vi "Read I16 analogue Data.vi"(6 "Block Header":string, 7 "Channel info":T1[](array[typedef]), 8 "Time Trace In":T2[](array[typedef]), 9 "Anaologue Index":i32[](array[numeric]), 10 "pos offset (bytes:0)":i32, 11 "refnum":refnum<file>) -> (0 "Time Trace out":T2[](array[typedef]), 1 "EOF?":bool, 2 "mark after read (bytes)":i32)   [LabVIEW 2017]
uses:
  Controls/Time_Trace_Cluster.ctl
  Controls/Read I16 data cluster.ctl
  Globals/Meas_global.vi
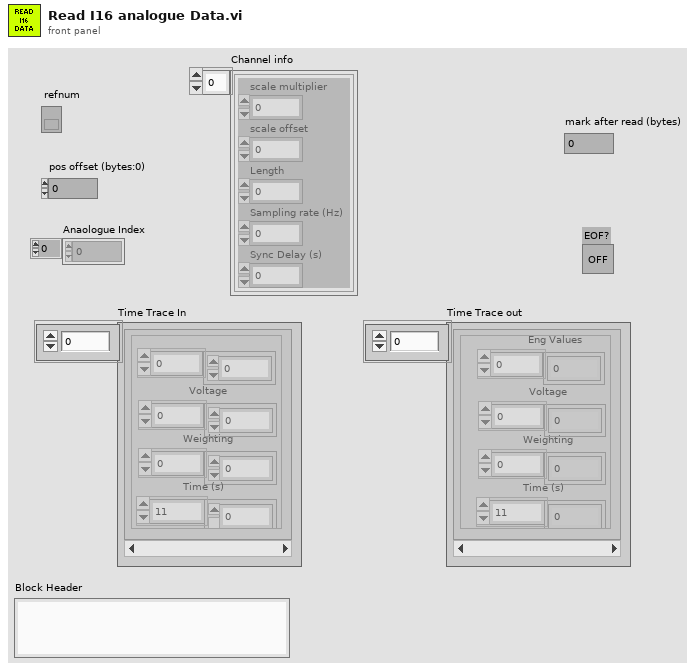
[diagram p1: front panel]
types:
  T1 = typedef "Read I16 data cluster.ctl" = cluster{"scale multiplier":dbl, "scale offset":dbl, "Length":i32, "Sampling rate (Hz)":dbl, "Sync Delay (s)":dbl}
  T2 = typedef "Time_Trace_Cluster.ctl" = cluster{"Weighting":dbl[], "Time (s)":dbl[], "Voltage":dbl[], "Eng Values":dbl[]}
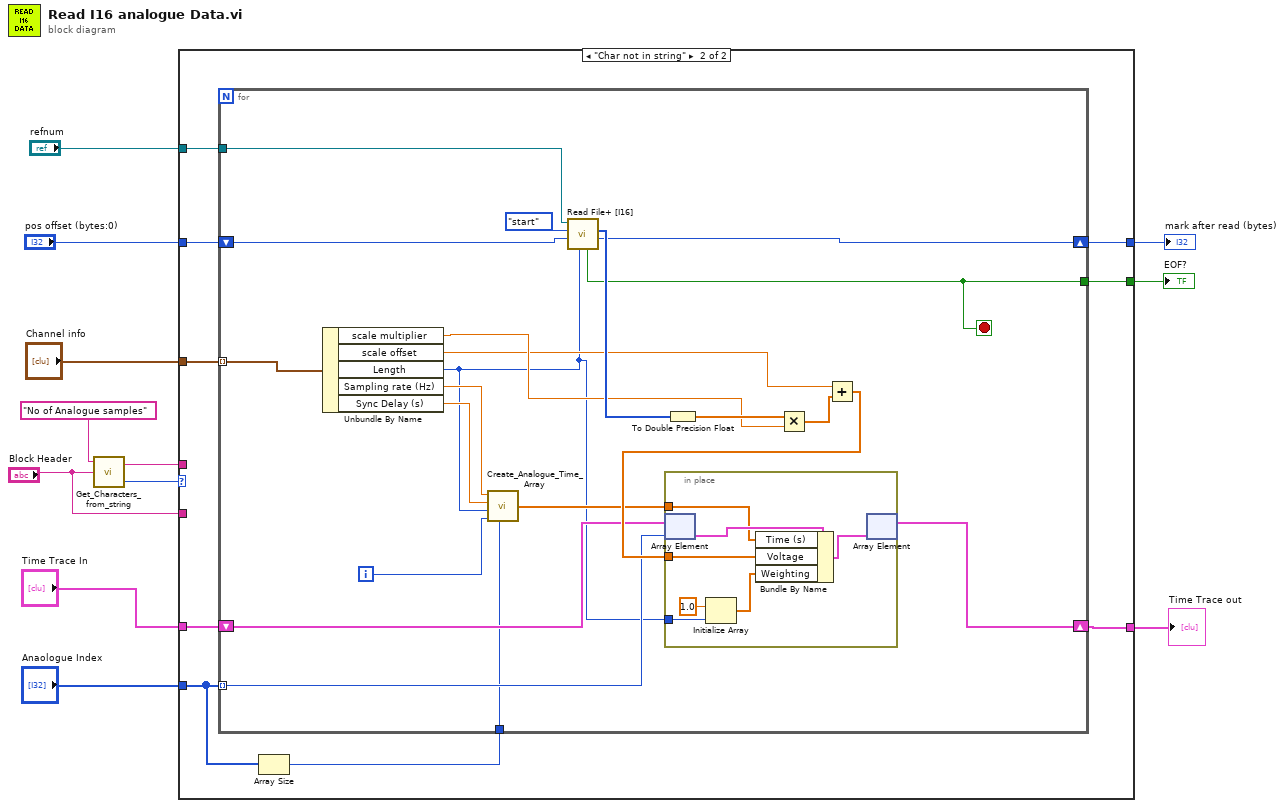
[diagram p0: block diagram]
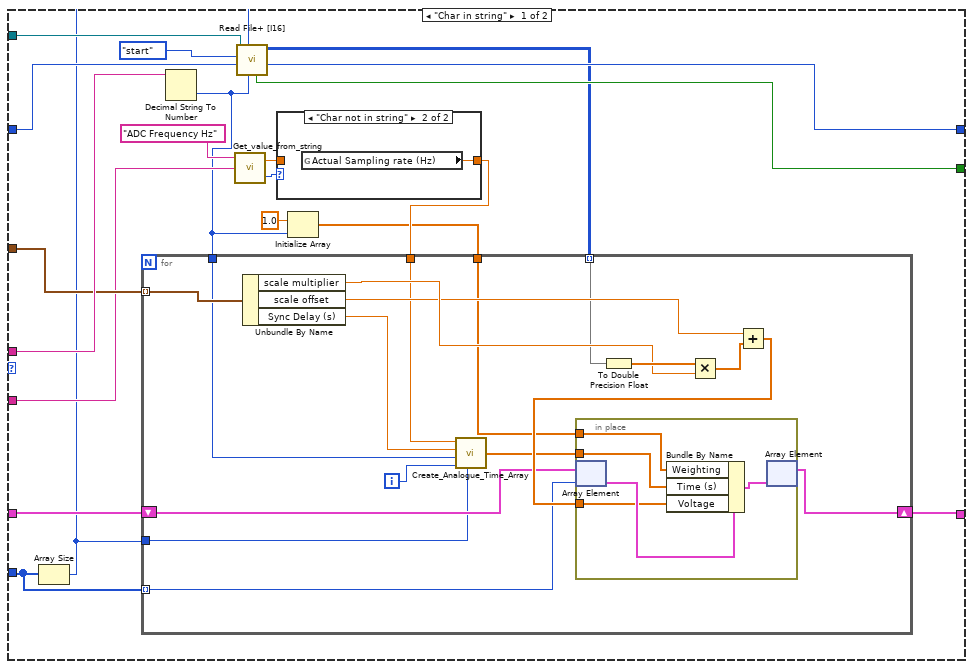
[diagram p2: hidden frame]
diagram:
  n1 = call "Get_Characters_from_string.vi"("Input string"="Block Header", "Variable name"="No of Analogue samples") -> ("Status"=w4:enum16{"Char in string", "Char not in string"}, "Value"=w3:string)  [unwired: 1 in]
  n2 = case shown="\"Char not in string\"" w4 {
    tunnel: "Time Trace In" -> [w23 w65]
    tunnel: "Anaologue Index" -> [w21 w58]
    tunnel: "Channel info" -> [w19 w64]
    tunnel: [w22 w63] -> w9
    tunnel: "pos offset (bytes:0)" -> [w28 w62]
    tunnel: [w27 w61] -> w7
    tunnel: "refnum" -> [w26 w60]
    tunnel: w3 -> [w25 _]
    tunnel: [w24 w59] -> w2
    tunnel: "Block Header" -> [w18 _]
    frame "Char in string" {
      n3 = Array Size(array=w21) -> (size(s)=w16:i32)
      n4 = Decimal String To Number(string=w25) -> (number=w14:i32)  [unwired: 3 out]
      n5 = call "Get_value_from_string.vi"("Input string"=w18, "Variable name"="ADC Frequency Hz") -> ("Status"=w31:enum16{"Char in string", "Char not in string"}, "Value"=w32:dbl)  [unwired: 1 in]
      n6 = call <vilib>:"Read File+ [I16].vi"("2D number of columns/1D count"=w14, "2D number of rows"=w16, "pos offset (bytes:0)"=w28, "pos mode (rel. to current:2)"=enum16{"start", "end", "current"}."start", "refnum"=w26) -> ("mark after read (bytes)"=w27:i32, "2D data"=w20:i16[][], "EOF?"=w24:bool)  [unwired: 1 in, 3 out]
      n7 = case shown="\"Char not in string\"" w31 {
        tunnel: w32 -> [w55 _]
        tunnel: [w55 w56] -> w17
        frame "Char in string" {
        }
        frame "Char not in string" {
          n8 = global read "Meas_global.vi" "Actual Sampling rate (Hz)"() -> (w56:dbl)
        }
      }
      n9 = Initialize Array(1.0 ("element"), w14) -> (w13:dbl[])
      n10 = for {
        shift-right: [w43] -> w22
        shift-left: w23 -> [w44]
        tunnel: w21 -> [w42] mode=indexing
        tunnel: w20 -> [w41] mode=indexing
        tunnel: w19 -> [w40] mode=indexing
        tunnel: w14 -> [w39]
        tunnel: w17 -> [w38]
        tunnel: w16 -> [w34]
        tunnel: w13 -> [w33]
        i -> [w35]
        n11 = Unbundle By Name(w40) -> ("scale multiplier"=w47:dbl, "scale offset"=w46:dbl, "Sync Delay (s)"=w36:dbl)
        n12 = call "Create_Analogue_Time_Array.vi"("Sampling Rate (Hz)"=w38, "Sync Delay (s)"=w36, "No of Samples"=w39, "Index"=w35, "No Of Analogue Chs"=w34) -> ("Times"=w37:dbl[])
        n13 = To Double Precision Float(number=w41) -> (double precision float=w48:dbl[])
        n14 = Multiply(x=w48, y=w47) -> (x*y=w49:dbl[])
        n15 = Add(x=w46, y=w49) -> (x+y=w45:dbl[])
        n16 = in-place {
          in-place-border: w45 -> [w53]
          in-place-border: w37 -> [w51]
          in-place-border: w33 -> [w50]
          n17 = in-place-array #1(w44, w42) -> (w54:T2)
          n18 = Bundle By Name(cluster=w54, "Weighting"=w50, "Time (s)"=w51, "Voltage"=w53) -> (w52:T2)
          n19 = in-place-array #1(w52) -> (w43:T2[])  [unwired: 1 out]
        }
      }
    }
    frame "Char not in string" {
      n20 = Array Size(array=w58) -> (size(s)=w57:i32)
      n21 = for {
        shift-right: [w78] -> w63
        shift-left: w65 -> [w79]
        tunnel: w58 -> [w77] mode=indexing
        tunnel: w64 -> [w76] mode=indexing
        shift-right: [w74] -> w61
        shift-left: w62 -> [w75]
        tunnel: w60 -> [w71]
        tunnel: [w70] -> w59
        tunnel: w57 -> [w67]
        i -> [w68]
        stop <- w70 stop-if-true
        n22 = Unbundle By Name(w76) -> ("scale multiplier"=w82:dbl, "scale offset"=w81:dbl, "Length"=w66:i32, "Sampling rate (Hz)"=w73:dbl, "Sync Delay (s)"=w69:dbl)
        n23 = call "Create_Analogue_Time_Array.vi"("Sampling Rate (Hz)"=w73, "Sync Delay (s)"=w69, "No of Samples"=w66, "Index"=w68, "No Of Analogue Chs"=w67) -> ("Times"=w72:dbl[])
        n24 = call <vilib>:"Read File+ [I16].vi"("2D number of columns/1D count"=w66, "pos offset (bytes:0)"=w75, "pos mode (rel. to current:2)"=enum16{"start", "end", "current"}."start", "refnum"=w71) -> ("mark after read (bytes)"=w74:i32, "1D data"=w83:i16[], "EOF?"=w70:bool)  [unwired: 2 in, 3 out]
        n25 = To Double Precision Float(number=w83) -> (double precision float=w84:dbl[])
        n26 = Multiply(x=w84, y=w82) -> (x*y=w85:dbl[])
        n27 = Add(x=w81, y=w85) -> (x+y=w80:dbl[])
        n28 = in-place {
          in-place-border: w80 -> [w92]
          in-place-border: w72 -> [w90]
          in-place-border: w66 -> [w89]
          n29 = in-place-array #2(w79, w77) -> (w93:T2)
          n30 = Initialize Array(1.0 ("element"), w89) -> (w87:dbl[])
          n31 = Bundle By Name(cluster=w93, "Time (s)"=w90, "Voltage"=w92, "Weighting"=w87) -> (w91:T2)
          n32 = in-place-array #2(w91) -> (w78:T2[])  [unwired: 1 out]
        }
      }
    }
  }
  "Time Trace out" <- w9
  "mark after read (bytes)" <- w7
  "EOF?" <- w2
